vi "DMM_Get Attributes.vi"(8 "error in (no error)":errorcluster, 11 "DMM Virtual in":refnum<class "DMM Virtual.lvclass">) -> (0 "error out":errorcluster, 2 "Class Attributes":T1, 3 "DMM Virtual out":refnum<class "DMM Virtual.lvclass">)   [LabVIEW 2018, in "DMM Virtual.lvclass"]
uses:
  DMM Virtual.lvclass
  Controls/Class Attributes Cluster.ctl
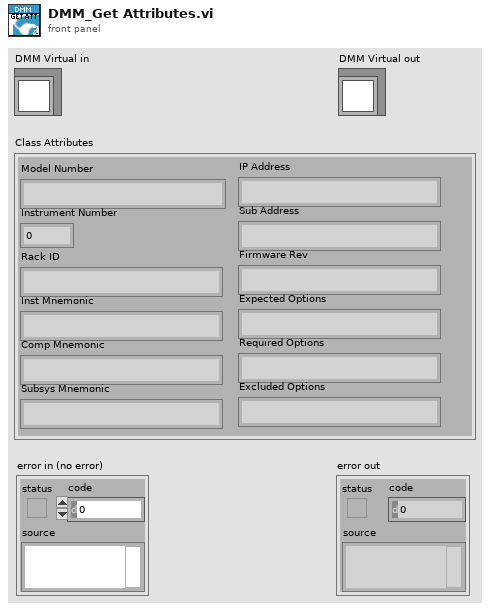
[diagram p1: front panel]
types:
  T1 = typedef "Class Attributes Cluster.ctl" = cluster{"Model Number":string, "Instrument Number":u8, "Rack ID":string, "Inst Mnemonic":string, "Comp Mnemonic":string, "Subsys Mnemonic":string, "IP Address":string, "Sub Address":string, "Firmware Rev":string, "Expected Options":string, "Required Options":string, "Excluded Options":string}
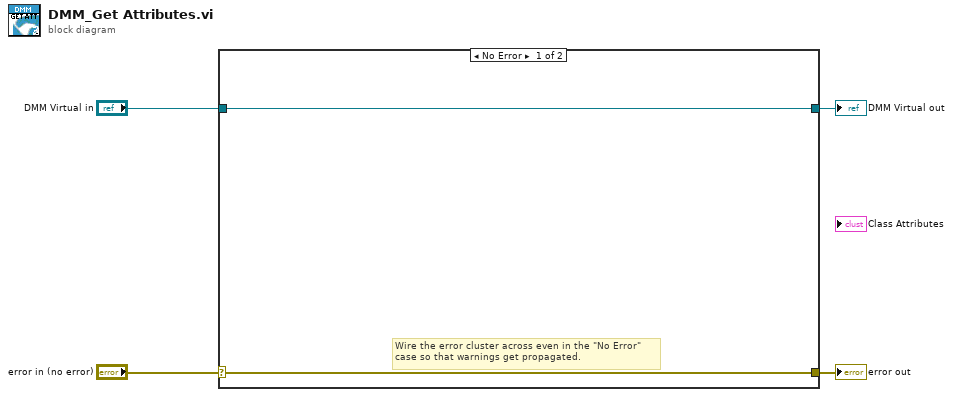
[diagram p0: block diagram]
diagram:
  n1 = case shown="No Error" "error in (no error)" {
    selector: "error in (no error)" -> [w5 w8]
    tunnel: [w5 w8] -> w3
    tunnel: [w6 w7] -> w1
    tunnel: "DMM Virtual in" -> [w6 w7]
    frame No Error {
      # "Wire the error cluster across even in the \"No Error\"\ncase so that warnings get propagated."
    }
    frame Error {
    }
  }
  "error out" <- w3
  "DMM Virtual out" <- w1
